vi "Check Response.vi"(8 "error in (no error)":errorcluster, 10 "output cluster in":T1) -> (0 "error out":errorcluster, 2 "output cluster out":T1)   [LabVIEW 2020]
uses:
  Data Cluster.ctl
  <vilib>/Utility/miscctls.llb/LVDateTimeRec.ctl
panel:
  out "NumSamples":u8
  out "Samples (new, old, older)":u8[](array[numeric]) format="%02x"
  out "Status":u8
  out "Offset":u8
  out "Range":u8
  out "Sample (new)":sgl
  out "Sample (old)":sgl
  out "Sample (older)":sgl
  out "Mo":sgl
  out "unsigned byte array":u8[](array[numeric])
  out "Mf":sgl
  # "Send Data:"
  # "Receive Data:"
  # "Send Data:"
  # "Receive Data:"
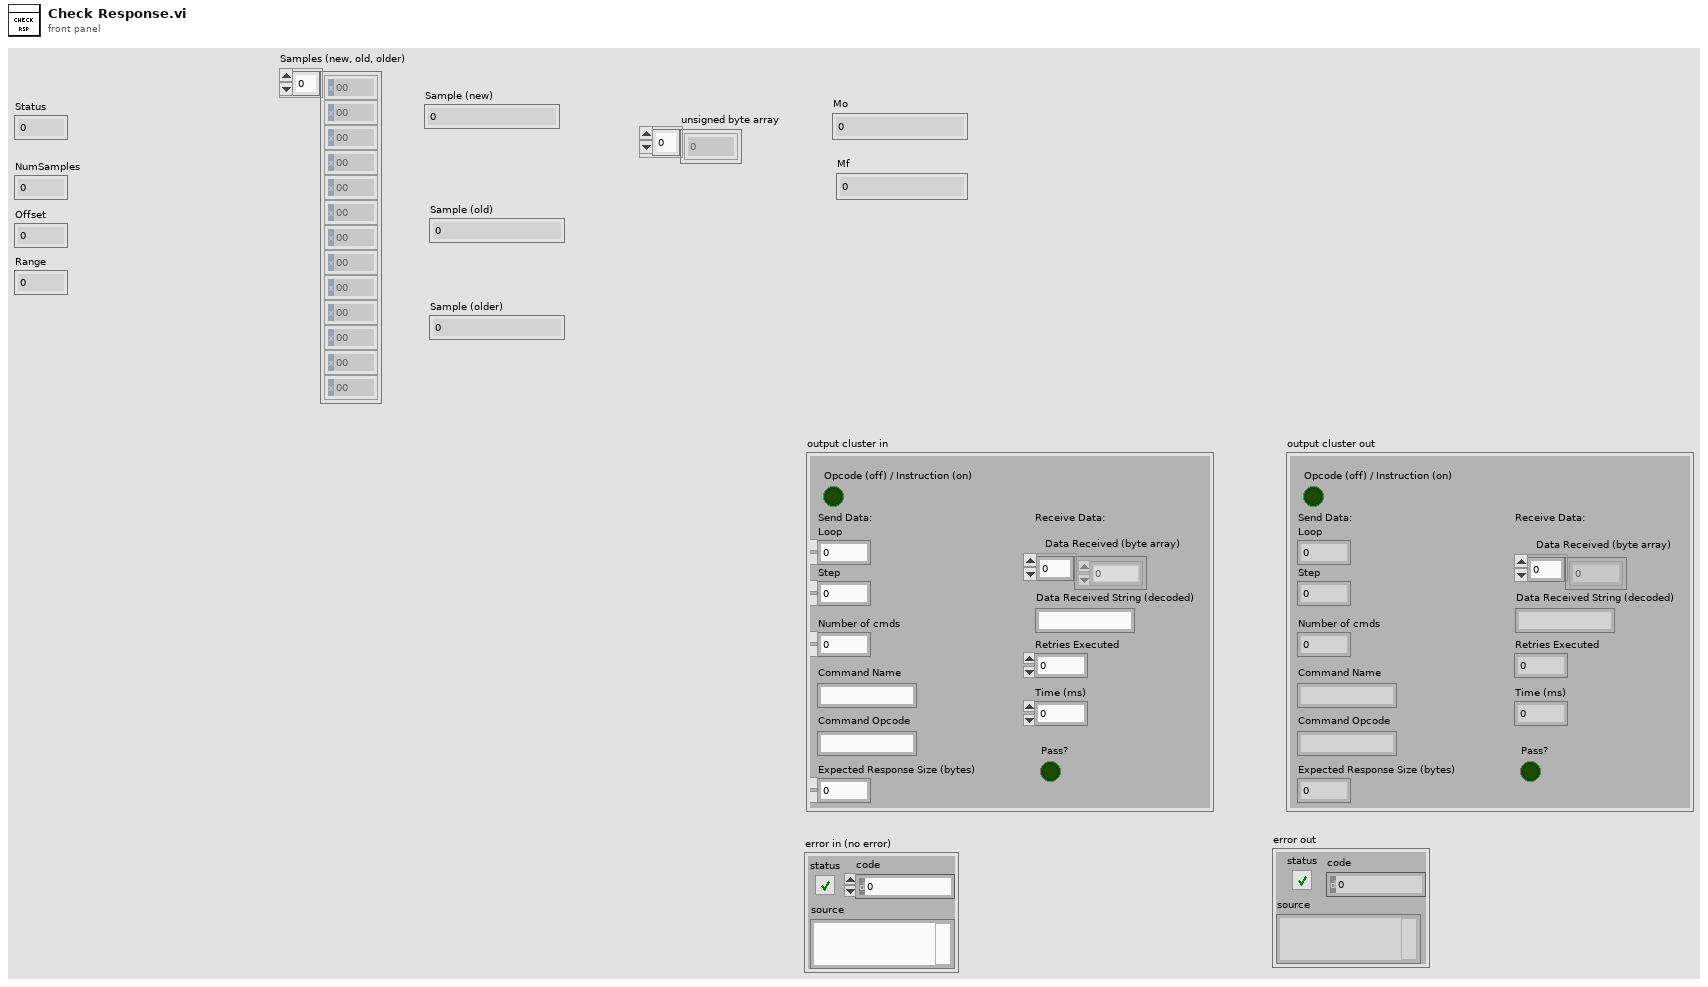
[diagram p1: front panel]
types:
  T1 = typedef "Data Cluster.ctl" = cluster{"Command Name":string, "Command Opcode ":string, "Step":dbl, "Loop":dbl, "Expected Response Size (bytes)":u16, "Number of cmds":dbl, "Data Received (byte array)":u8[], "Retries Executed":u16, "Time (ms)":u16, "Pass?":bool, "Opcode (off) / Instruction (on)":bool, "Data Received String (decoded)":string}
  T2 = typedef "LVDateTimeRec.ctl" = cluster{"fractional second":dbl, "second":i32, "minute":i32, "hour":i32, "day of month":i32, "month":i32, "year":i32, "day of week":i32, "day of year":i32, "DST":i32}
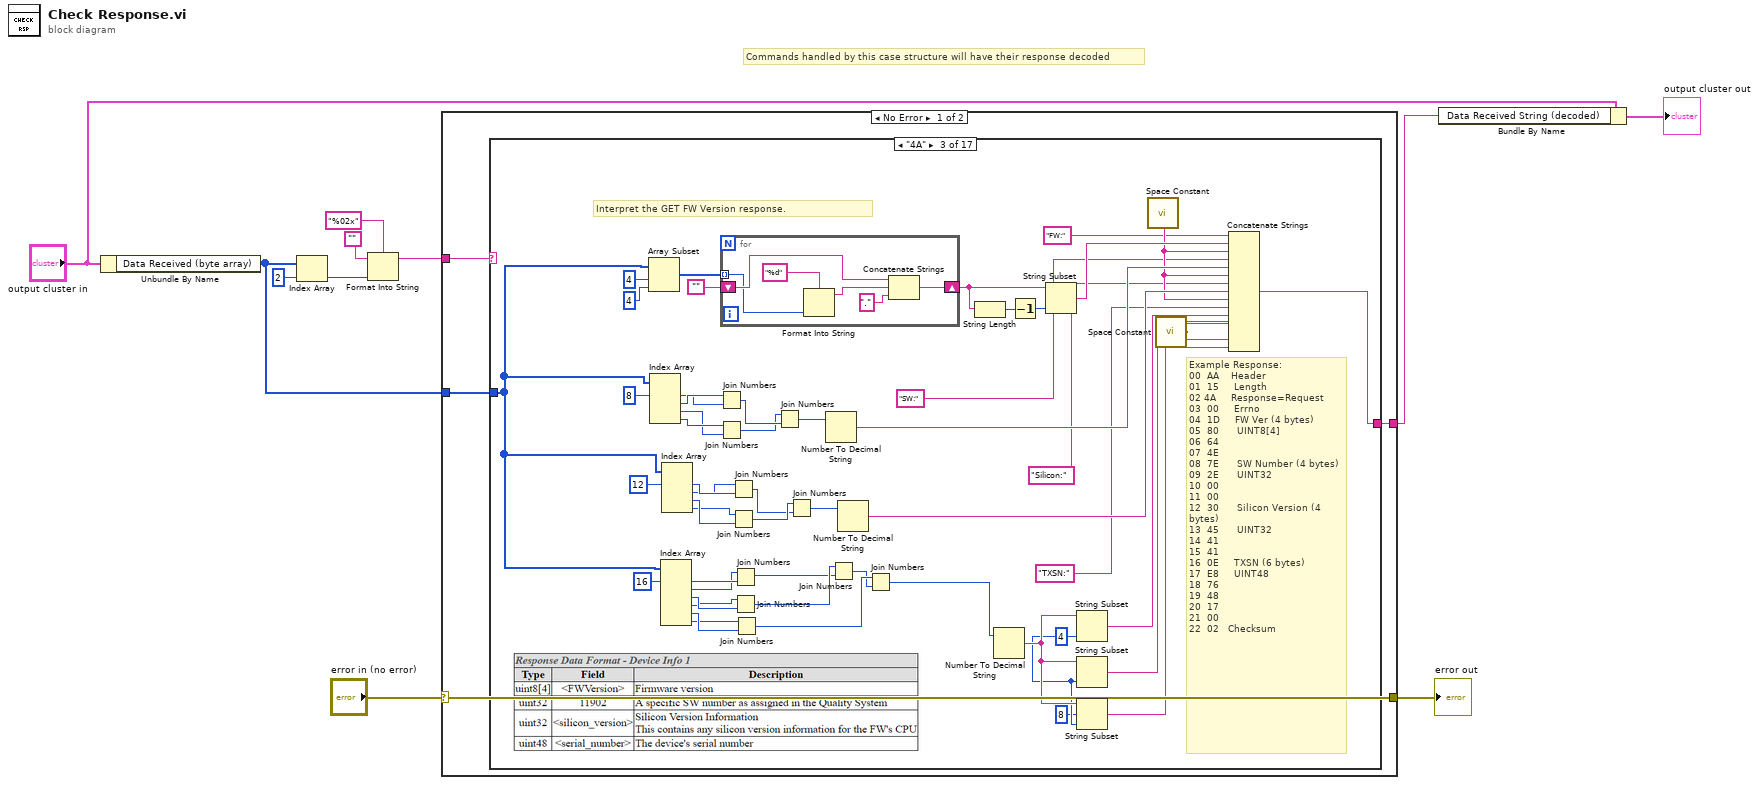
[diagram p0: block diagram]
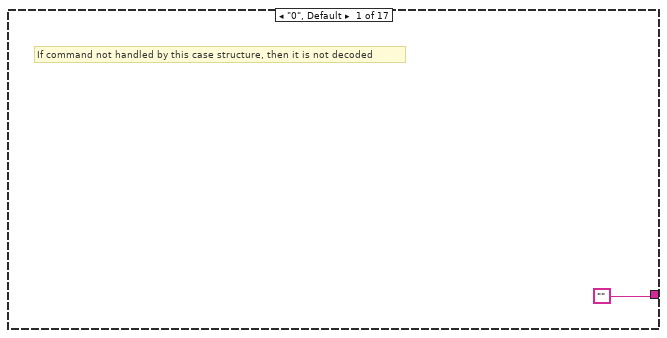
[diagram p2: hidden frame]
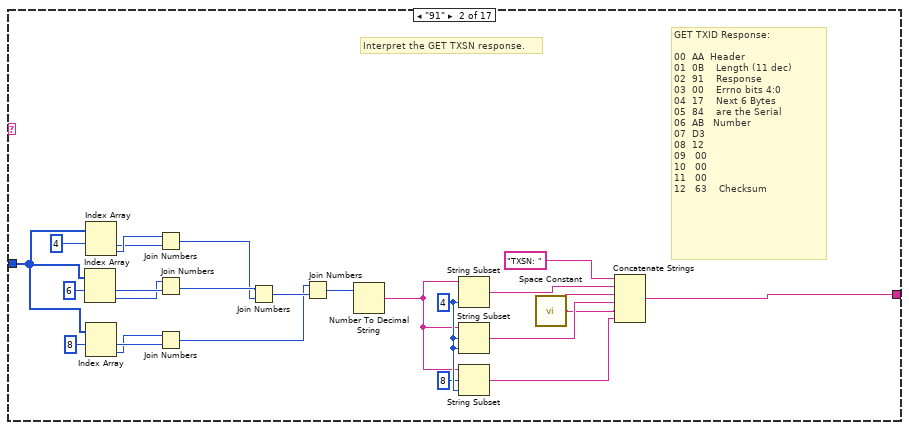
[diagram p3: hidden frame]
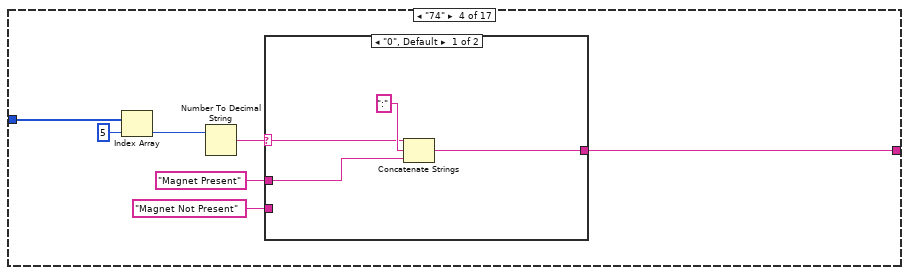
[diagram p4: hidden frame]
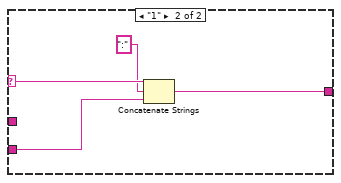
[diagram p5: hidden frame]
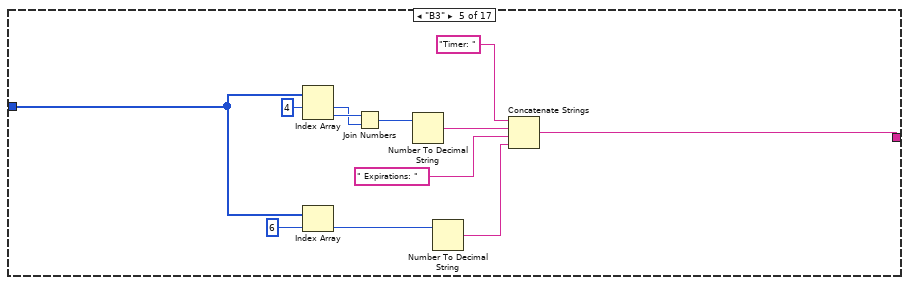
[diagram p6: hidden frame]
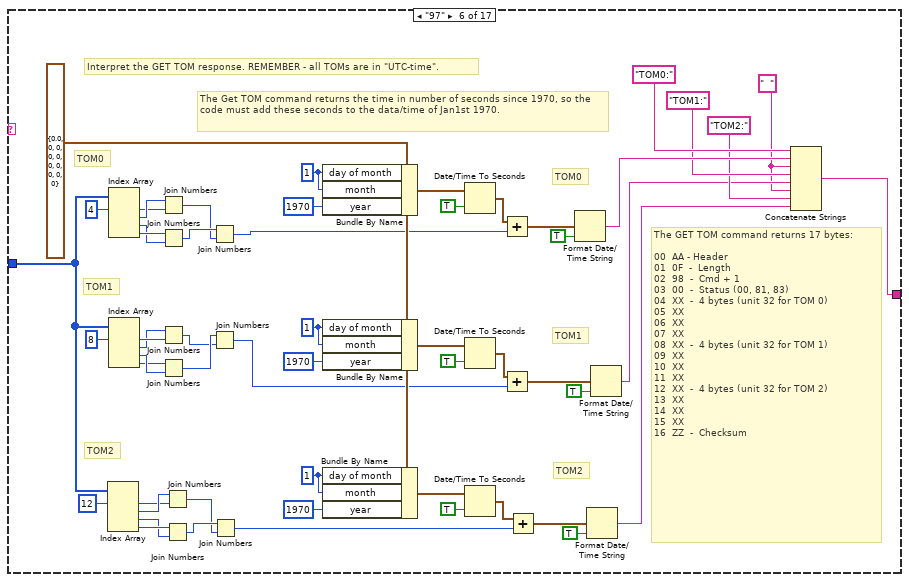
[diagram p7: hidden frame]
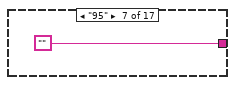
[diagram p8: hidden frame]
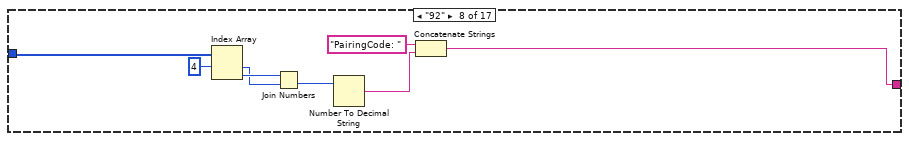
[diagram p9: hidden frame]
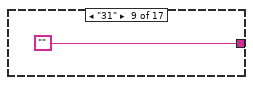
[diagram p10: hidden frame]
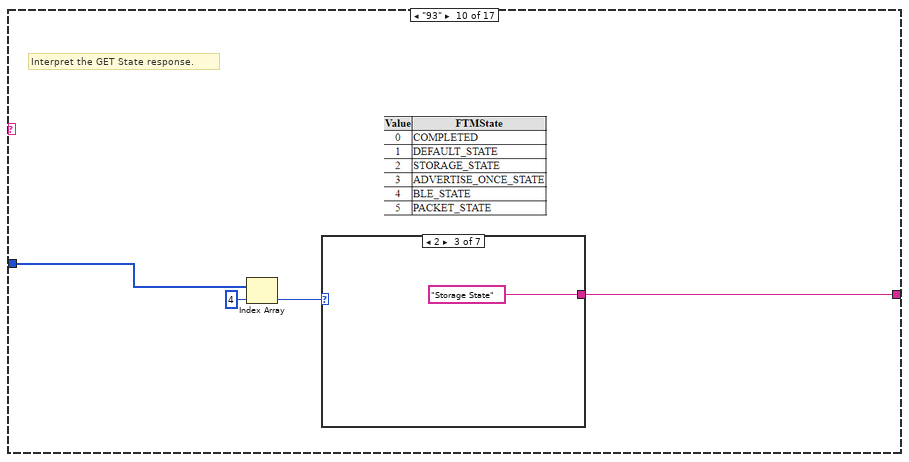
[diagram p11: hidden frame]
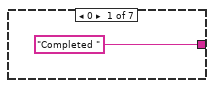
[diagram p12: hidden frame]
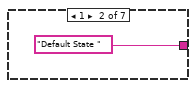
[diagram p13: hidden frame]
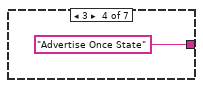
[diagram p14: hidden frame]
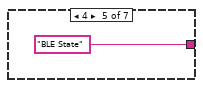
[diagram p15: hidden frame]
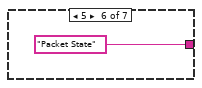
[diagram p16: hidden frame]
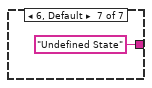
[diagram p17: hidden frame]
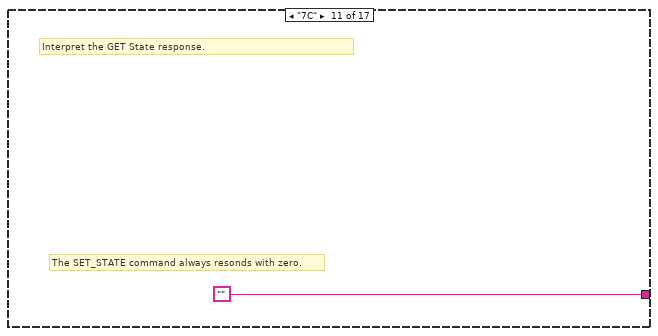
[diagram p18: hidden frame]
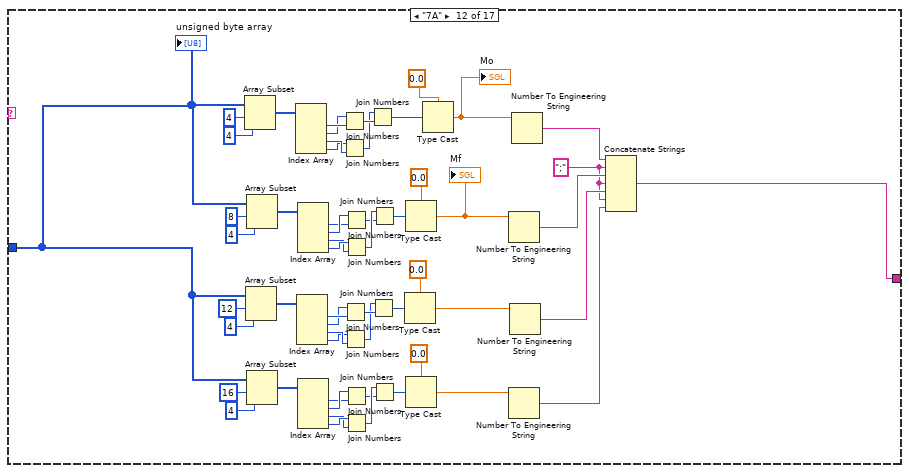
[diagram p19: hidden frame]
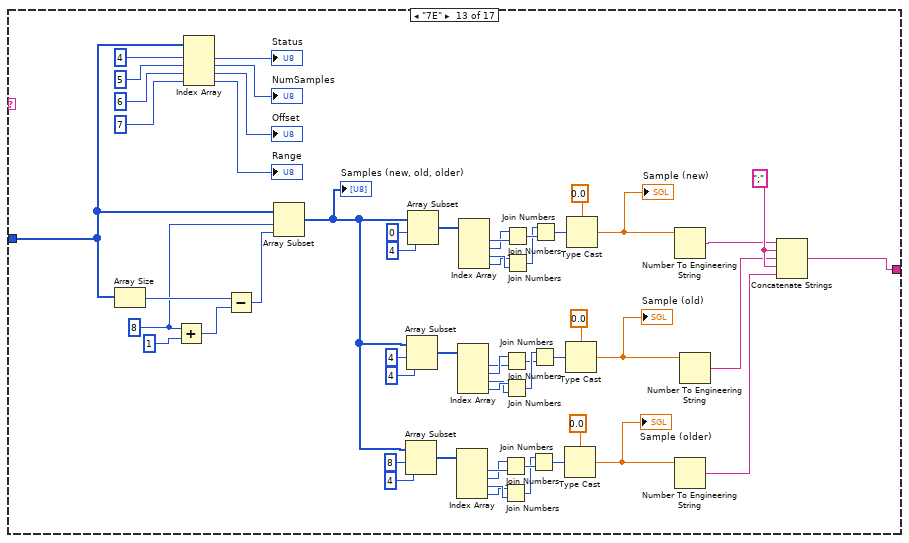
[diagram p20: hidden frame]
diagram:
  # "Commands handled by this case structure will have their response decoded"
  n1 = Unbundle By Name("output cluster in") -> ("Data Received (byte array)"=w4:u8[])
  n2 = Index Array(array=w4, index=2) -> (element=w8:u8)
  n3 = Format Into String(format string="%02x", initial string="", w8) -> (resulting string=w7:string)  [unwired: 1 in, 1 out]
  n4 = case shown="No Error" "error in (no error)" {
    selector: "error in (no error)" -> [w13 w361]
    tunnel: w4 -> [w15 _]
    tunnel: [w14 ""] -> w2
    tunnel: [w13 w361] -> w5
    tunnel: w7 -> [w12 _]
    frame No Error {
      n5 = case shown="\"4A\"" w12 {
        tunnel: w15 -> [_ w34 w56 w104 w115 w133 _ w186 _ w192 _ w208 w259 w318 w338 w350 _]
        tunnel: ["" w30 w55 w99 w116 w132 "" w182 "" w191 "" w231 w258 w317 w329 w348 ""] -> w14
        frame "0", Default {
          # "If command not handled by this case structure, then it is not decoded"
        }
        frame "91" {
          w23 = 4 ("length (rest)")
          # "GET TXID Response:\n\n00  AA  Header\n01  0B    Length (11 dec)\n02  91    Response\n03  00    Errno bits 4:0\n04  17    Next 6 Bytes \n05  84    are the Serial\n06  AB   Number\n07  D3\n08  12\n09   00\n10   00\n11   00\n12   63    Checksum"
          # "Interpret the GET TXSN response."
          n6 = Index Array(array=w34, index #1=6 ("index")) -> (element #1=w32:u8, element #2=w31:u8)  [unwired: 1 in]
          n7 = Index Array(array=w34, index #1=4 ("index")) -> (element #1=w38:u8, element #2=w39:u8)  [unwired: 1 in]
          n8 = Index Array(array=w34, index #1=8 ("index")) -> (element #1=w35:u8, element #2=w33:u8)  [unwired: 1 in]
          n9 = Join Numbers(hi=w39, lo=w38) -> ((hi.lo)=w27:u16)
          n10 = Join Numbers(hi=w31, lo=w32) -> ((hi.lo)=w28:u16)
          n11 = Join Numbers(hi=w33, lo=w35) -> ((hi.lo)=w25:u16)
          n12 = Join Numbers(hi=w28, lo=w27) -> ((hi.lo)=w26:u32)
          n13 = Join Numbers(hi=w25, lo=w26) -> ((hi.lo)=w24:u64)
          n14 = Number To Decimal String(number=w24) -> (decimal integer string=w21:string)  [unwired: 1 in]
          n15 = String Subset(string=w21, length (rest)=w23) -> (substring=w20:string)  [unwired: 1 in]
          n16 = String Subset(string=w21, offset (0)=w23, length (rest)=w23) -> (substring=w19:string)
          n17 = String Subset(string=w21, offset (0)=8, length (rest)=w23) -> (substring=w17:string)
          n18 = call <vilib>:"Space Constant.vi"() -> ("String"=w18:string)
          n19 = Concatenate Strings("TXSN: " ("String"), w20, w18, w19, w18, w17) -> (w30:string)
        }
        frame "4A" {
          w68 = 4 ("length (rest)")
          # "Example Response:\n00  AA    Header\n01  15     Length\n02 4A     Response=Request\n03  00     Errno\n04  1D     FW Ver (4 bytes)   \n05  80      UINT8[4]\n06  64    \n07  4E    \n08  7E      SW Number (4 bytes)\n09  2E      UINT32\n10  00\n11  00\n12  30      Silicon Version (4 bytes)\n13  45      UINT32\n14  41\n15  41     \n16  0E     TXSN (6 bytes)\n17  E8     UINT48\n18  76    \n19  48\n20  17\n21  00\n22  02   Checksum"
          # "Interpret the GET FW Version response."
          n20 = Array Subset(array=w56, index=4, length=4) -> (w74:u8[])
          n21 = Index Array(array=w56, index #1=8 ("index")) -> (element #1=w53:u8, element #2=w54:u8, element #3=w51:u8, element #4=w52:u8)  [unwired: 3 in]
          n22 = Index Array(array=w56, index #1=16 ("index")) -> (element #1=w46:u8, element #2=w45:u8, element #3=w44:u8, element #4=w43:u8, element #5=w42:u8, element #6=w41:u8)  [unwired: 5 in]
          n23 = Index Array(array=w56, index #1=12 ("index")) -> (element #1=w50:u8, element #2=w49:u8, element #3=w48:u8, element #4=w47:u8)  [unwired: 3 in]
          n24 = Join Numbers(hi=w54, lo=w53) -> ((hi.lo)=w76:u16)
          n25 = Join Numbers(hi=w52, lo=w51) -> ((hi.lo)=w75:u16)
          n26 = for {
            tunnel: w74 -> [w93] mode=indexing
            shift-right: [w95] -> w73
            shift-left: "" -> [w97]
            n27 = Format Into String(format string="%d", w93) -> (resulting string=w96:string)  [unwired: 2 in, 1 out]
            n28 = Concatenate Strings(w97, w96, "." ("string")) -> (w95:string)
          }
          n29 = Join Numbers(hi=w49, lo=w50) -> ((hi.lo)=w80:u16)
          n30 = Join Numbers(hi=w47, lo=w48) -> ((hi.lo)=w81:u16)
          n31 = Join Numbers(hi=w45, lo=w46) -> ((hi.lo)=w88:u16)
          n32 = Join Numbers(hi=w43, lo=w44) -> ((hi.lo)=w89:u16)
          n33 = Join Numbers(hi=w41, lo=w42) -> ((hi.lo)=w91:u16)
          n34 = Join Numbers(hi=w75, lo=w76) -> ((hi.lo)=w77:u32)
          n35 = Join Numbers(hi=w81, lo=w80) -> ((hi.lo)=w79:u32)
          n36 = Number To Decimal String(number=w77) -> (decimal integer string=w78:string)  [unwired: 1 in]
          n37 = Join Numbers(hi=w89, lo=w88) -> ((hi.lo)=w90:u32)
          n38 = Number To Decimal String(number=w79) -> (decimal integer string=w82:string)  [unwired: 1 in]
          n39 = Join Numbers(hi=w91, lo=w90) -> ((hi.lo)=w92:u64)
          n40 = String Length(string=w73) -> (length=w72:i32)
          n41 = Number To Decimal String(number=w92) -> (decimal integer string=w87:string)  [unwired: 1 in]
          n42 = Decrement(x=w72) -> (x-1=w71:i32)
          n43 = String Subset(string=w73, length (rest)=w71) -> (substring=w70:string)  [unwired: 1 in]
          n44 = String Subset(string=w87, length (rest)=w68) -> (substring=w84:string)  [unwired: 1 in]
          n45 = String Subset(string=w87, offset (0)=w68, length (rest)=w68) -> (substring=w85:string)
          n46 = String Subset(string=w87, offset (0)=8, length (rest)=w68) -> (substring=w86:string)
          n47 = call <vilib>:"Space Constant.vi"() -> ("String"=w69:string)
          n48 = call <vilib>:"Space Constant.vi"() -> ("String"=w83:string)
          n49 = Concatenate Strings("FW:", w70, w69, "SW:", w78, w69, "Silicon:", w82, w69, "TXSN:", w84, w83, w85, w83, w86) -> (w55:string)
        }
        frame "74" {
          n50 = Index Array(array=w104, index=5) -> (element=w103:u8)
          n51 = Number To Decimal String(number=w103) -> (decimal integer string=w102:string)  [unwired: 1 in]
          n52 = case shown="\"0\", Default" w102 {
            selector: w102 -> [w108 w113]
            tunnel: "Magnet Not Present" -> [_ w111]
            tunnel: "Magnet Present" -> [w107 _]
            tunnel: [w106 w110] -> w99
            frame "0", Default {
              n53 = Concatenate Strings(w108, ":", w107) -> (w106:string)
            }
            frame "1" {
              n54 = Concatenate Strings(w113, ":", w111) -> (w110:string)
            }
          }
        }
        frame "B3" {
          n55 = Index Array(array=w115, index #1=4 ("index")) -> (element #1=w123:u8, element #2=w124:u8)  [unwired: 1 in]
          n56 = Index Array(array=w115, index=6) -> (element=w122:u8)
          n57 = Join Numbers(hi=w124, lo=w123) -> ((hi.lo)=w125:u16)
          n58 = Number To Decimal String(number=w125) -> (decimal integer string=w118:string)  [unwired: 1 in]
          n59 = Number To Decimal String(number=w122) -> (decimal integer string=w117:string)  [unwired: 1 in]
          n60 = Concatenate Strings("Timer: " ("string"), w118, " Expirations: " ("string"), w117) -> (w116:string)
        }
        frame "97" {
          w126 = "  "
          w148 = 1 ("day of month")
          w151 = 1 ("day of month")
          w158 = 1 ("day of month")
          w144 = T2 {"fractional second"=0.0, "second"=0, "minute"=0, "hour"=0, "day of month"=0, "month"=0, "year"=0, "day of week"=0, "day of year"=0, "DST"=0} ("date time rec")
          # "TOM2"
          # "TOM1"
          # "TOM0"
          # "TOM2"
          # "TOM1"
          # "TOM0"
          # "Interpret the GET TOM response. REMEMBER - all TOMs are in \"UTC-time\"."
          # "The GET TOM command returns 17 bytes:\n\n00  AA - Header\n01  0F  -  Length\n02  98  -  Cmd + 1\n03  00  -  Status (00, 81, 83)\n04  XX  -  4 bytes (unit 32 for TOM 0)\n05  XX\n06  XX\n07  XX\n08  XX  -  4 bytes (unit 32 for TOM 1)\n09  XX\n10  XX\n11  XX\n12  XX  -  4 bytes (unit 32 for TOM 2)\n13  XX\n14  XX\n15  XX\n16  ZZ  -  Checksum"
          # "The Get TOM command returns the time in number of seconds since 1970, so the code must add these seconds to the data/time of Jan1st 1970."
          n61 = Index Array(array=w133, index #1=12 ("index")) -> (element #1=w168:u8, element #2=w169:u8, element #3=w166:u8, element #4=w167:u8)  [unwired: 3 in]
          n62 = Index Array(array=w133, index #1=4 ("index")) -> (element #1=w178:u8, element #2=w179:u8, element #3=w176:u8, element #4=w177:u8)  [unwired: 3 in]
          n63 = Index Array(array=w133, index #1=8 ("index")) -> (element #1=w173:u8, element #2=w172:u8, element #3=w175:u8, element #4=w174:u8)  [unwired: 3 in]
          n64 = Join Numbers(hi=w179, lo=w178) -> ((hi.lo)=w164:u16)
          n65 = Join Numbers(hi=w177, lo=w176) -> ((hi.lo)=w165:u16)
          n66 = Join Numbers(hi=w172, lo=w173) -> ((hi.lo)=w162:u16)
          n67 = Join Numbers(hi=w174, lo=w175) -> ((hi.lo)=w163:u16)
          n68 = Join Numbers(hi=w169, lo=w168) -> ((hi.lo)=w160:u16)
          n69 = Join Numbers(hi=w167, lo=w166) -> ((hi.lo)=w161:u16)
          n70 = Join Numbers(hi=w165, lo=w164) -> ((hi.lo)=w143:u32)
          n71 = Join Numbers(hi=w163, lo=w162) -> ((hi.lo)=w142:u32)
          n72 = Join Numbers(hi=w161, lo=w160) -> ((hi.lo)=w141:u32)
          n73 = Bundle By Name(cluster=w144, "day of month"=w158, "month"=w158, "year"=1970) -> (w159:T2)
          n74 = Bundle By Name(cluster=w144, "day of month"=w151, "month"=w151, "year"=1970) -> (w150:T2)
          n75 = Bundle By Name(cluster=w144, "day of month"=w148, "month"=w148, "year"=1970) -> (w149:T2)
          n76 = Date/Time To Seconds(1:TRUE ("is UTC (F)"), 2:w159) -> (0:w155:timestamp)
          n77 = Date/Time To Seconds(1:TRUE ("is UTC (F)"), 2:w150) -> (0:w154:timestamp)
          n78 = Date/Time To Seconds(1:TRUE ("is UTC (F)"), 2:w149) -> (0:w145:timestamp)
          n79 = Add(x=w155, y=w143) -> (x+y=w135:timestamp)
          n80 = Add(x=w154, y=w142) -> (x+y=w136:timestamp)
          n81 = Add(x=w145, y=w141) -> (x+y=w140:timestamp)
          n82 = Format Date/Time String(seconds (now)=w135, UTC format=TRUE) -> (date/time string=w134:string)  [unwired: 1 in]
          n83 = Format Date/Time String(seconds (now)=w140, UTC format=TRUE) -> (date/time string=w129:string)  [unwired: 1 in]
          n84 = Format Date/Time String(seconds (now)=w136, UTC format=TRUE) -> (date/time string=w127:string)  [unwired: 1 in]
          n85 = Concatenate Strings("TOM0:", w134, w126, "TOM1:", w127, w126, "TOM2:", w129) -> (w132:string)
        }
        frame "95" {
        }
        frame "92" {
          n86 = Index Array(array=w186, index #1=4 ("index")) -> (element #1=w188:u8, element #2=w189:u8)  [unwired: 1 in]
          n87 = Join Numbers(hi=w189, lo=w188) -> ((hi.lo)=w185:u16)
          n88 = Number To Decimal String(number=w185) -> (decimal integer string=w184:string)  [unwired: 1 in]
          n89 = Concatenate Strings("PairingCode: " ("string"), w184) -> (w182:string)
        }
        frame "31" {
        }
        frame "93" {
          # "Interpret the GET State response."
          n90 = Index Array(array=w192, index=4) -> (element=w193:u8)
          n91 = case shown="2" w193 {
            tunnel: ["Completed " "Default State " "Storage State" "Advertise Once State" "BLE State" "Packet State" "Undefined State"] -> w191
            frame 0 {
            }
            frame 1 {
            }
            frame 2 {
            }
            frame 3 {
            }
            frame 4 {
            }
            frame 5 {
            }
            frame 6, Default {
            }
          }
        }
        frame "7C" {
          # "The SET_STATE command always resonds with zero."
          # "Interpret the GET State response."
        }
        frame "7A" {
          w204 = ";"
          n92 = Array Subset(array=w208, index=4, length=4) -> (w247:u8[])
          n93 = Array Subset(array=w208, index=12, length=4) -> (w220:u8[])
          n94 = Array Subset(array=w208, index=8, length=4) -> (w245:u8[])
          n95 = Array Subset(array=w208, index=16, length=4) -> (w219:u8[])
          n96 = Index Array(array=w247) -> (element #1=w255:u8, element #2=w254:u8, element #3=w253:u8, element #4=w252:u8)  [unwired: 4 in]
          n97 = Index Array(array=w220) -> (element #1=w228:u8, element #2=w227:u8, element #3=w226:u8, element #4=w225:u8)  [unwired: 4 in]
          n98 = Index Array(array=w245) -> (element #1=w237:u8, element #2=w238:u8, element #3=w239:u8, element #4=w240:u8)  [unwired: 4 in]
          n99 = Index Array(array=w219) -> (element #1=w211:u8, element #2=w212:u8, element #3=w213:u8, element #4=w214:u8)  [unwired: 4 in]
          n100 = Join Numbers(hi=w254, lo=w255) -> ((hi.lo)=w251:u16)
          n101 = Join Numbers(hi=w252, lo=w253) -> ((hi.lo)=w250:u16)
          n102 = Join Numbers(hi=w227, lo=w228) -> ((hi.lo)=w224:u16)
          n103 = Join Numbers(hi=w225, lo=w226) -> ((hi.lo)=w223:u16)
          n104 = Join Numbers(hi=w238, lo=w237) -> ((hi.lo)=w241:u16)
          n105 = Join Numbers(hi=w240, lo=w239) -> ((hi.lo)=w242:u16)
          n106 = Join Numbers(hi=w212, lo=w211) -> ((hi.lo)=w215:u16)
          n107 = Join Numbers(hi=w214, lo=w213) -> ((hi.lo)=w216:u16)
          n108 = Join Numbers(hi=w250, lo=w251) -> ((hi.lo)=w249:u32)
          n109 = Join Numbers(hi=w223, lo=w224) -> ((hi.lo)=w222:u32)
          n110 = Join Numbers(hi=w242, lo=w241) -> ((hi.lo)=w243:u32)
          n111 = Join Numbers(hi=w216, lo=w215) -> ((hi.lo)=w217:u32)
          n112 = Type Cast(type=sgl 0.0, x=w222) -> (*(type *) &x=w207:sgl)
          n113 = Type Cast(type=sgl 0.0, x=w243) -> (*(type *) &x=w234:sgl)
          "Mf" <- w234
          n114 = Type Cast(type=sgl 0.0, x=w217) -> (*(type *) &x=w206:sgl)
          n115 = Type Cast(type=sgl 0.0, x=w249) -> (*(type *) &x=w246:sgl)
          "Mo" <- w246
          n116 = Number To Engineering String(4:w234) -> (0:w232:string)  [unwired: 3 in]
          n117 = Number To Engineering String(4:w206) -> (0:w203:string)  [unwired: 3 in]
          n118 = Number To Engineering String(4:w207) -> (0:w205:string)  [unwired: 3 in]
          n119 = Number To Engineering String(4:w246) -> (0:w233:string)  [unwired: 3 in]
          n120 = Concatenate Strings(w233, w204, w232, w204, w205, w204, w203) -> (w231:string)
          "unsigned byte array" <- w208
        }
        frame "7E" {
          w263 = ";"
          w311 = 8 ("index")
          n121 = Array Size(array=w259) -> (size(s)=w312:i32)
          n122 = Add(x=w311, y=1) -> (x+y=w309:i32)
          n123 = Index Array(array=w259, index #1=4 ("index"), index #2=5 ("index"), index #3=6 ("index"), index #4=7 ("index")) -> (element #1=→"Status":u8, element #2=→"NumSamples":u8, element #3=→"Offset":u8, element #4=→"Range":u8)
          n124 = Subtract(x=w312, y=w309) -> (x-y=w308:i32)
          n125 = Array Subset(array=w259, index=w311, length=w308) -> (w269:u8[])
          "Samples (new, old, older)" <- w269
          n126 = Array Subset(array=w269, index=8, length=4) -> (w270:u8[])
          n127 = Array Subset(array=w269, index=4, length=4) -> (w291:u8[])
          n128 = Array Subset(array=w269, index=0, length=4) -> (w292:u8[])
          n129 = Index Array(array=w270) -> (element #1=w278:u8, element #2=w277:u8, element #3=w276:u8, element #4=w275:u8)  [unwired: 4 in]
          n130 = Index Array(array=w291) -> (element #1=w283:u8, element #2=w284:u8, element #3=w285:u8, element #4=w286:u8)  [unwired: 4 in]
          n131 = Index Array(array=w292) -> (element #1=w300:u8, element #2=w299:u8, element #3=w298:u8, element #4=w297:u8)  [unwired: 4 in]
          n132 = Join Numbers(hi=w277, lo=w278) -> ((hi.lo)=w274:u16)
          n133 = Join Numbers(hi=w275, lo=w276) -> ((hi.lo)=w273:u16)
          n134 = Join Numbers(hi=w284, lo=w283) -> ((hi.lo)=w287:u16)
          n135 = Join Numbers(hi=w286, lo=w285) -> ((hi.lo)=w288:u16)
          n136 = Join Numbers(hi=w299, lo=w300) -> ((hi.lo)=w296:u16)
          n137 = Join Numbers(hi=w297, lo=w298) -> ((hi.lo)=w295:u16)
          n138 = Join Numbers(hi=w273, lo=w274) -> ((hi.lo)=w272:u32)
          n139 = Join Numbers(hi=w288, lo=w287) -> ((hi.lo)=w289:u32)
          n140 = Join Numbers(hi=w295, lo=w296) -> ((hi.lo)=w294:u32)
          n141 = Type Cast(type=sgl 0.0, x=w272) -> (*(type *) &x=w264:sgl)
          "Sample (older)" <- w264
          n142 = Type Cast(type=sgl 0.0, x=w289) -> (*(type *) &x=w265:sgl)
          "Sample (old)" <- w265
          n143 = Type Cast(type=sgl 0.0, x=w294) -> (*(type *) &x=w266:sgl)
          "Sample (new)" <- w266
          n144 = Number To Engineering String(4:w266) -> (0:w262:string)  [unwired: 3 in]
          n145 = Number To Engineering String(4:w264) -> (0:w260:string)  [unwired: 3 in]
          n146 = Number To Engineering String(4:w265) -> (0:w261:string)  [unwired: 3 in]
          n147 = Concatenate Strings(w262, w263, w261, w263, w260) -> (w258:string)
        }
        frame "22" {
          # "Interpret the GET Battery Voltages response."
          # "Voltages: Satatic, Dynamic"
          n148 = Index Array(array=w318, index #1=4 ("index")) -> (element #1=w326:u8, element #2=w325:u8)  [unwired: 1 in]
          n149 = Index Array(array=w318, index #1=6 ("index")) -> (element #1=w328:u8, element #2=w327:u8)  [unwired: 1 in]
          n150 = Join Numbers(hi=w325, lo=w326) -> ((hi.lo)=w322:u16)
          n151 = Join Numbers(hi=w327, lo=w328) -> ((hi.lo)=w321:u16)
          n152 = Number To Decimal String(number=w322) -> (decimal integer string=w320:string)  [unwired: 1 in]
          n153 = Number To Decimal String(number=w321) -> (decimal integer string=w315:string)  [unwired: 1 in]
          n154 = Concatenate Strings("Static:" ("string"), w320, "  ", "Dynamic:" ("string"), w315) -> (w317:string)
        }
        frame "C2" {
          # "Interpret the GET Temperature response."
          # "This is a bitmask of enabled and detected temperature sensors."
          # "Get Temp Response Format:\n\nAA  -  Header\n08    -  Length \nC3   -  Response (C2+1)\n00   -  Tx Status\n57    -  Bit-masked Temp Status (57 desired)\nD0   -  centi-degrees C (4 bytes) unit 32\n08\n00\n00 \n44   -  Checksum"
          # "Temp"
          # "Status (should be 0x57)"
          n155 = Index Array(array=w338, index #1=4 ("index")) -> (element #1=w335:u8, element #2=w337:u8, element #3=w344:u8)  [unwired: 2 in]
          n156 = Join Numbers(hi=w344, lo=w337) -> ((hi.lo)=w342:u16)
          n157 = Divide(x=w342, y=u16 100) -> (x/y=w340:dbl)
          n158 = Format Into String(format string="%02x", w335) -> (resulting string=w331:string)  [unwired: 2 in, 1 out]
          n159 = Number To Fractional String(number=w340, precision (6)=i16 2) -> (F-format string=w334:string)  [unwired: 2 in]
          n160 = Concatenate Strings("Temp:" ("string"), w334, "   ", "Status:" ("string"), w331) -> (w329:string)
        }
        frame "56" {
          # "Interpret the GET Battery Type response."
          n161 = Index Array(array=w350, index=6) -> (element=w347:u8)
          n162 = Number To Decimal String(number=w347) -> (decimal integer string=w346:string)  [unwired: 1 in]
          n163 = case shown="\"0\", Default" w346 {
            tunnel: ["Panasonic" "Murata" "Invalid" "Invalid" "Maxell" "Invalid" "Invalid"] -> w345
            frame "5" {
            }
            frame "6" {
            }
            frame "0", Default {
            }
            frame "1" {
            }
            frame "2" {
            }
            frame "3" {
            }
            frame "4" {
            }
          }
          n164 = Concatenate Strings("Type:", w345) -> (w348:string)
        }
        frame "4D" {
          # "The SET_STATE command has no response text."
          # "0x4E: Convert the Switch from CGM to FTM Mode (0x4D) Response"
        }
      }
    }
    frame Error {
    }
  }
  "error out" <- w5
  n165 = Bundle By Name(cluster="output cluster in", "Data Received String (decoded)"=w2) -> (→"output cluster out":T1)
